vi "Read data.vi"(8 "error in (no error)":errorcluster, 11 "Exit in":refnum<class "Exit.lvclass">) -> (0 "error out":errorcluster, 2 "data":cluster{"Socket":i32, "Info":string}, 3 "Exit out":refnum<class "Exit.lvclass">)   [LabVIEW 2019, in "SignalProcessing.lvlib" / "Exit.lvclass"]
uses:
  Exit.lvclass
  Exit.lvclass/Exit.ctl
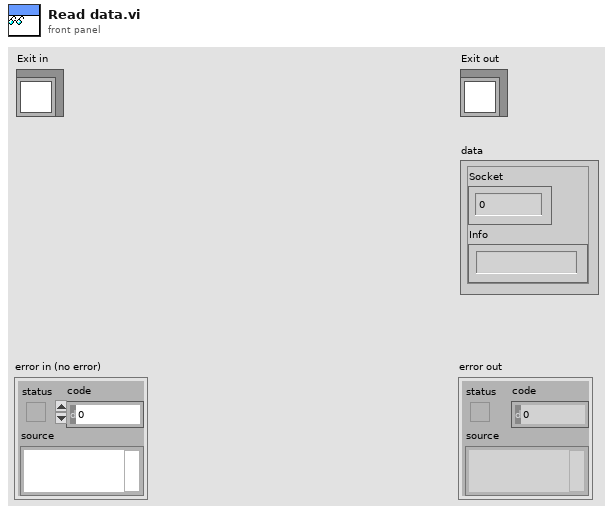
[diagram p1: front panel]
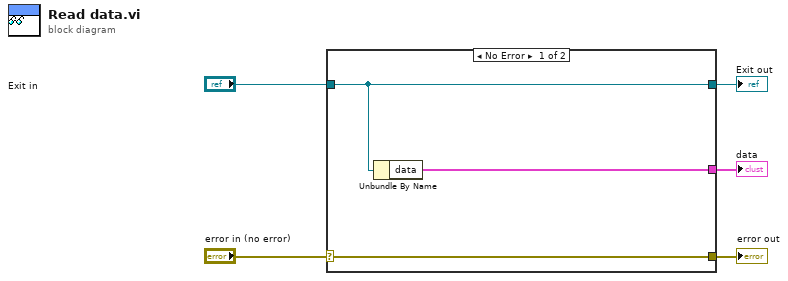
[diagram p0: block diagram]
diagram:
  n1 = case shown="No Error" "error in (no error)" {
    selector: "error in (no error)" -> [w8 w9]
    tunnel: [w8 w9] -> w4
    tunnel: [w7 w10] -> w2
    tunnel: "Exit in" -> [w7 w10]
    tunnel: [w6 _] -> w1
    frame No Error {
      n2 = Unbundle By Name(w7) -> ("data"=w6:cluster{"Socket":i32, "Info":string})
    }
    frame Error {
    }
  }
  "error out" <- w4
  "Exit out" <- w2
  "data" <- w1
